vi "GUI_BELLA_StageMegattentuator.vi"() -> ()   [LabVIEW 2020]
uses:
  Shared/GUI_Template/GUI_master/tcp_new_data_event.ctl
  Shared/GUI_Template/GUI_master/tcp new data cluster.ctl
panel:
  in  "Lock Control":bool
  in  "Change Position":bool
  out "Current Status":string
  in  "stop":bool
  in  "Position.Ch1::1":dbl=0.5 caption="Current Position" min=0.0 max=150.0 format="%_4f"
  out "error IO 2":errorcluster
  out "tcp data event":T1
  in  "GUIdevice 1":string="STAGE-LT-Megattenuator"
  in  "insert tag":bool=TRUE
  # "GUI_BELLA_StageMegattentuator"
  # "IN"
  # "OUT"
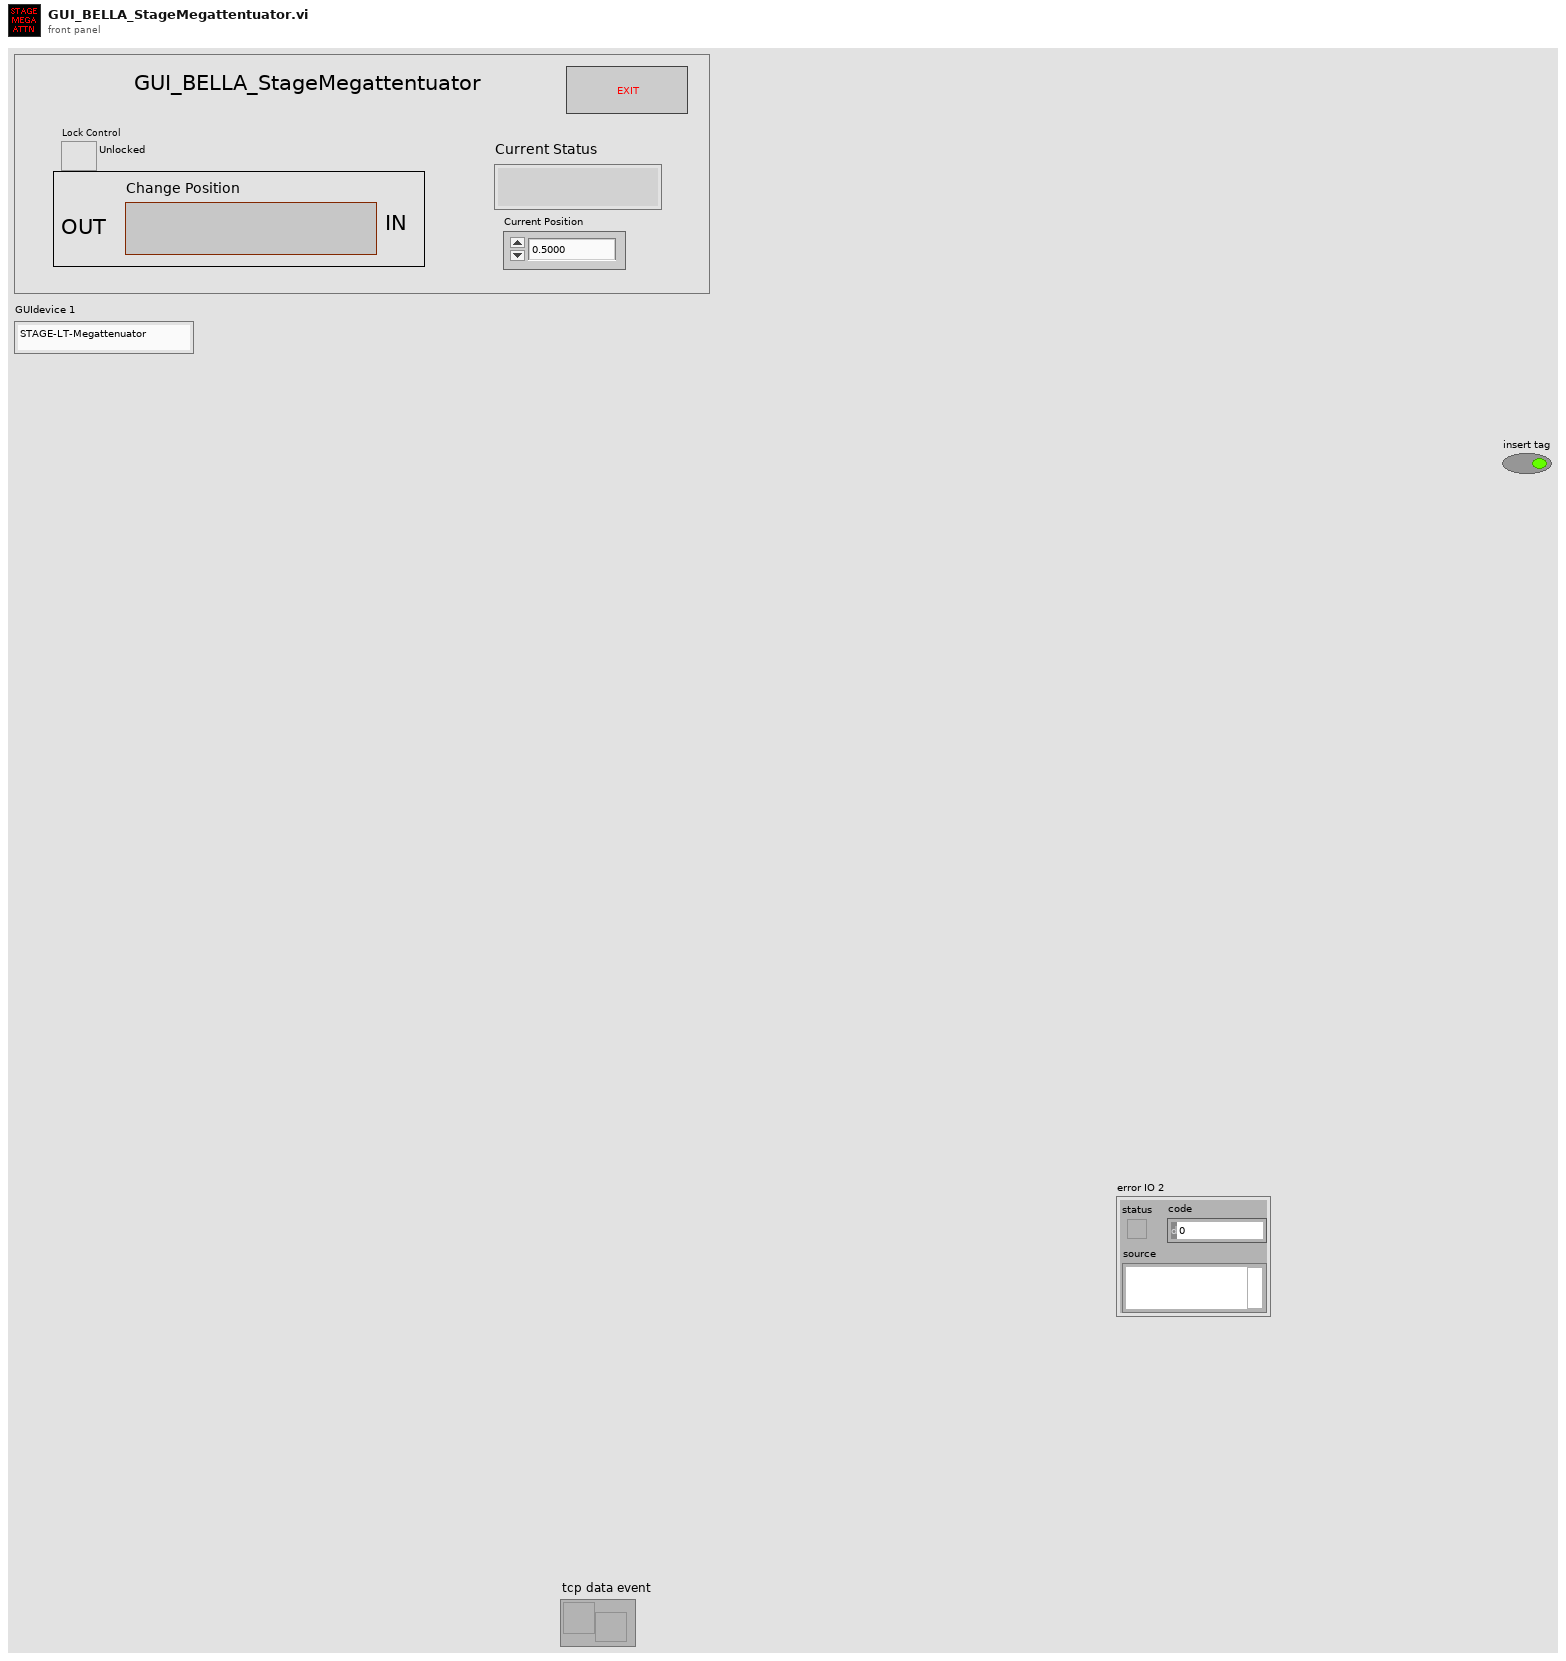
[diagram p1: front panel]
types:
  T1 = typedef "tcp_new_data_event.ctl" = refnum<user-event>
  T2 = typedef "tcp new data cluster.ctl" = cluster{"EventEnum":enum16{"new data", "connection status update"}, "Device name":string}
  T3 = enum8{"Enabled", "Disabled", "Disabled and Grayed Out"}
  T4 = enum32{"Invalid", "Standard", "Closed", "Hidden", "Minimized", "Maximized"}
  T5 = enum32{"invalid app kind", "Development System", "Run Time System", "Student Edition", "Embedded LabVIEW", "Evaluation", "Custom"}
  T6 = cluster{"Core":cluster{"Current VI Reference":refnum<vi>, "Close Panel on Exit?":bool}, "Your Boolean data":bool, "Your string data":string}
  T7 = cluster{"Current VI Reference":refnum<vi>, "Close Panel on Exit?":bool}
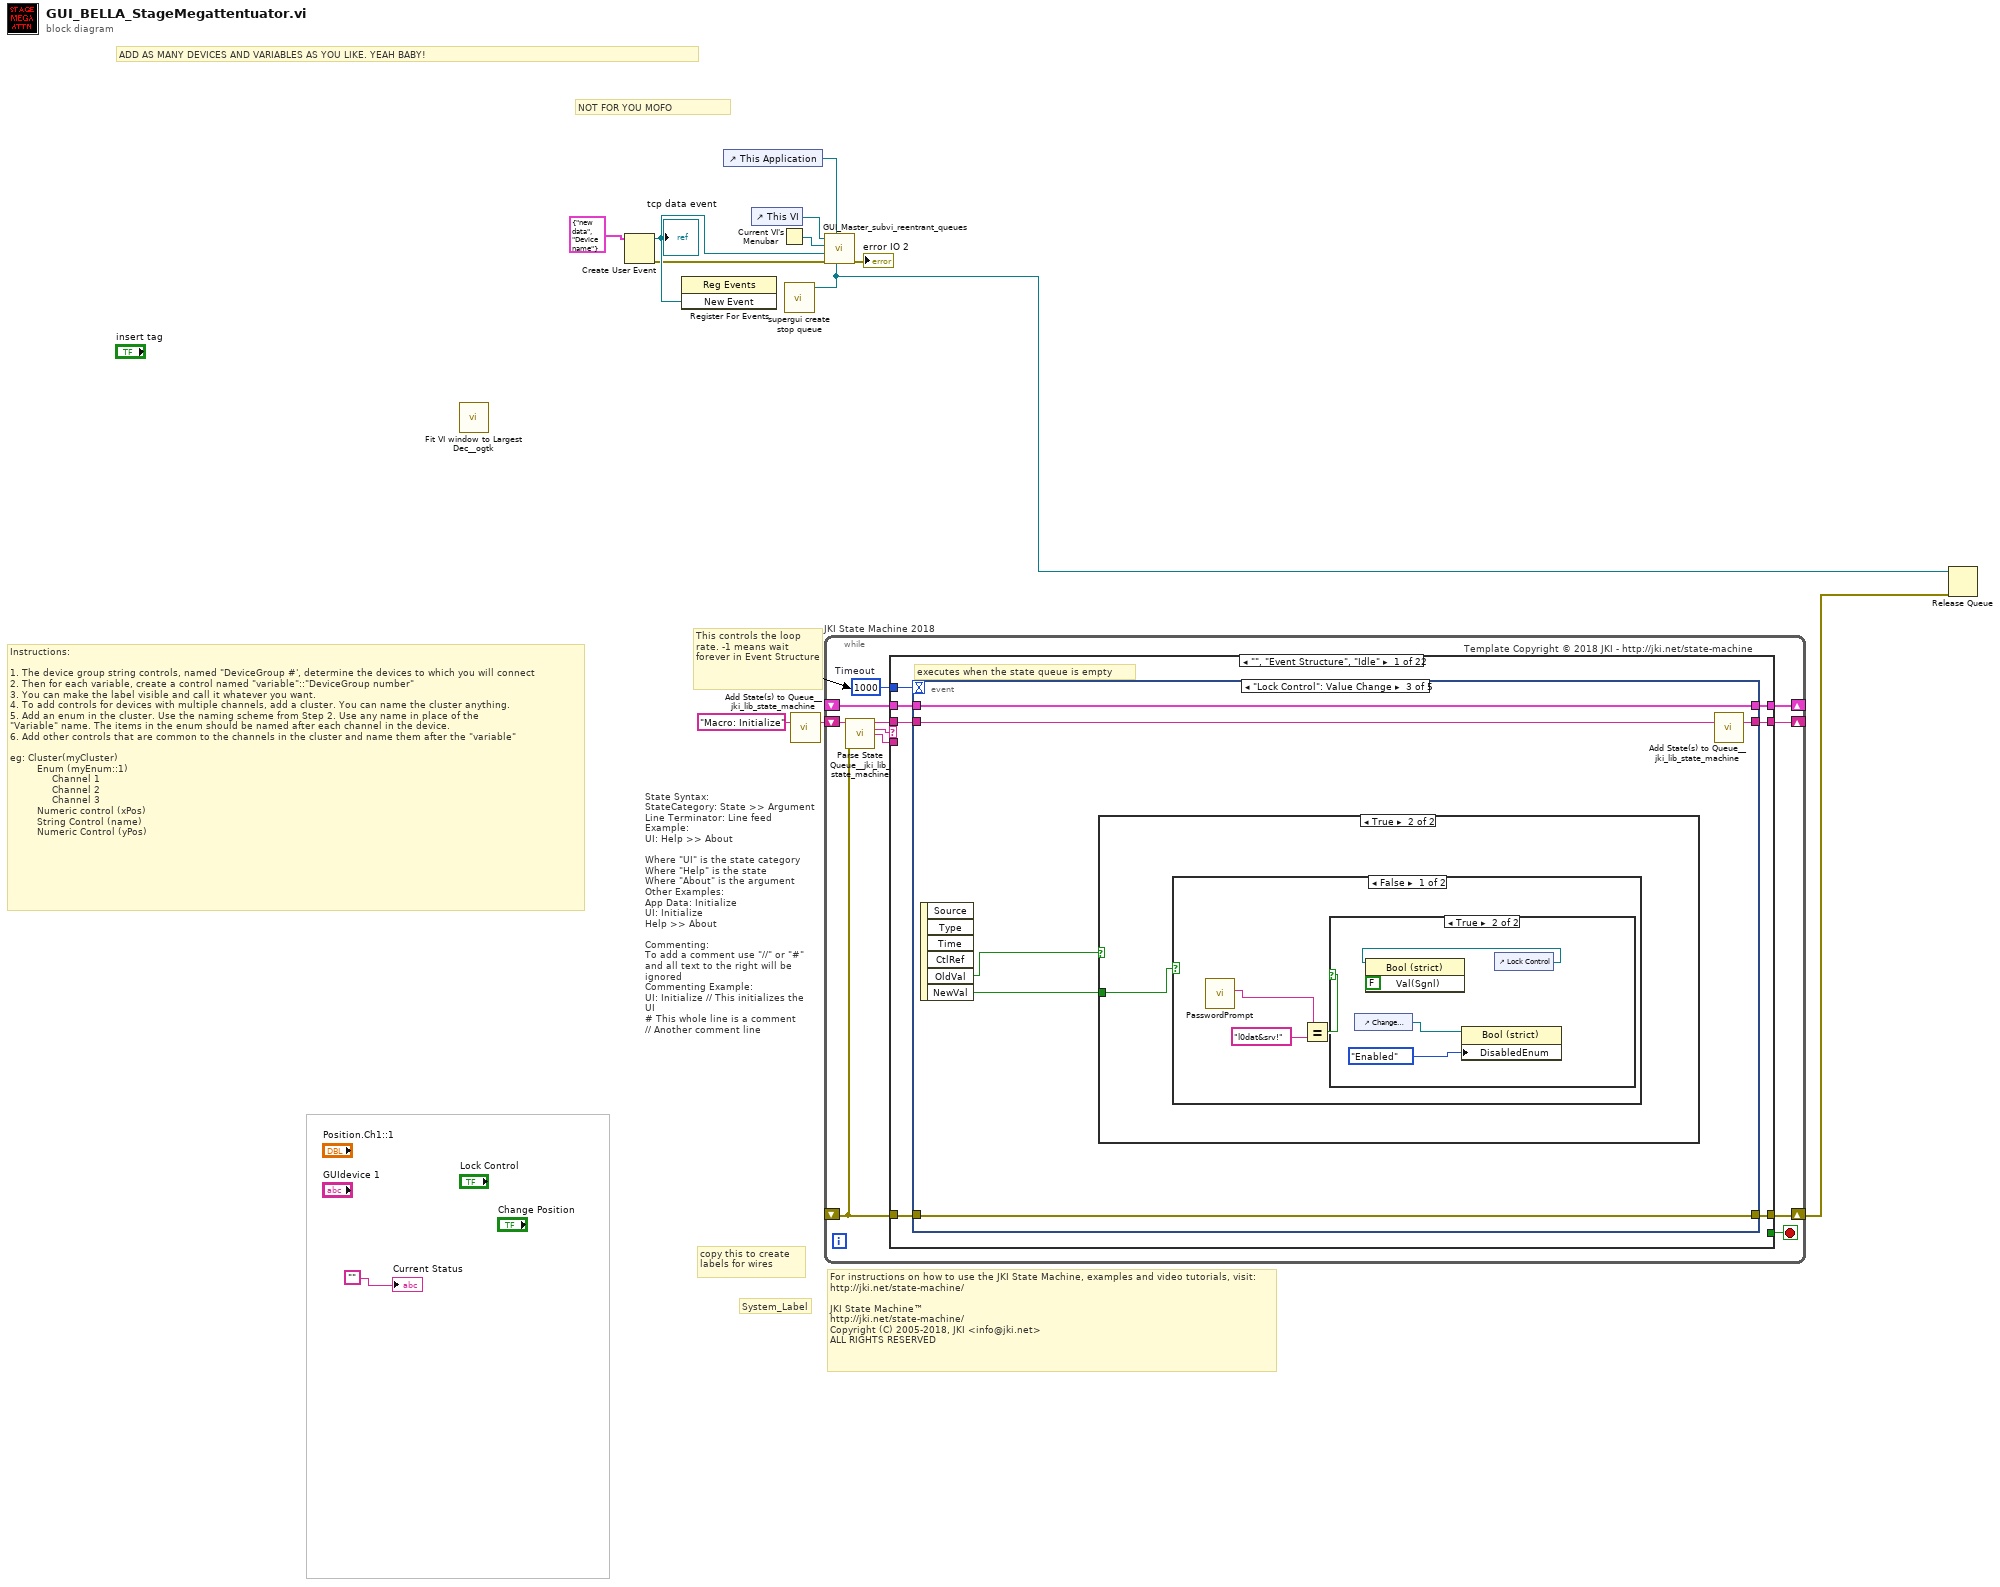
[diagram p0: block diagram]
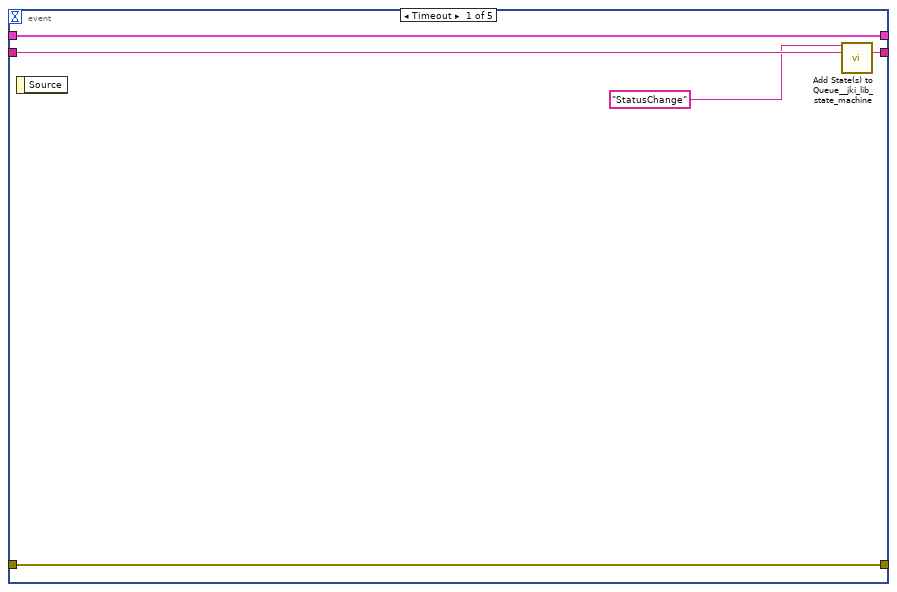
[diagram p2: hidden frame]
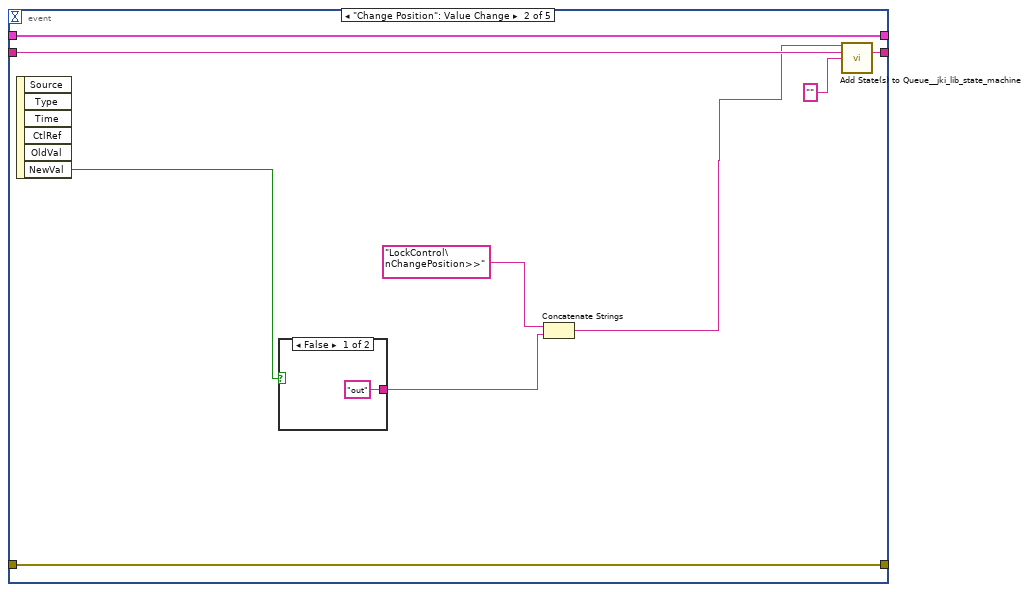
[diagram p3: hidden frame]
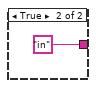
[diagram p4: hidden frame]
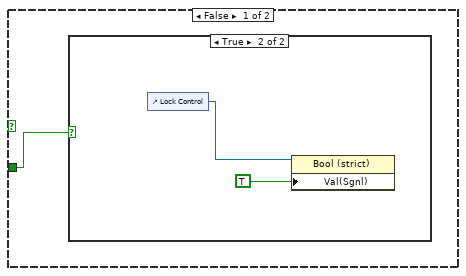
[diagram p5: hidden frame]
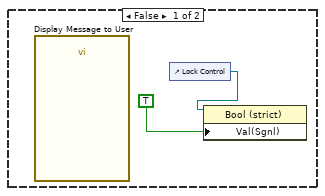
[diagram p7: hidden frame]
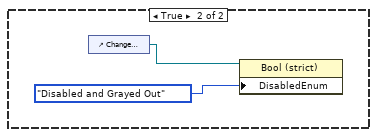
[diagram p8: hidden frame]
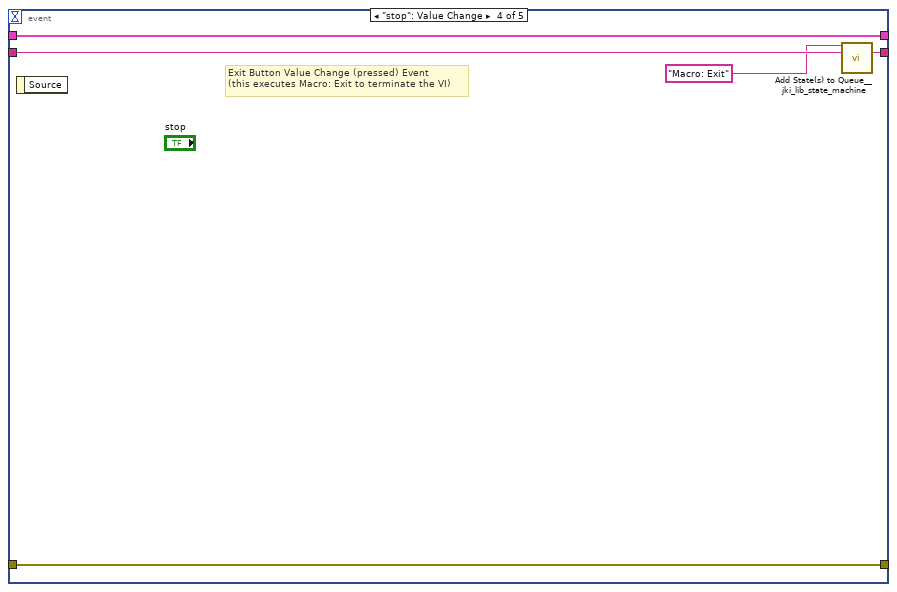
[diagram p9: hidden frame]
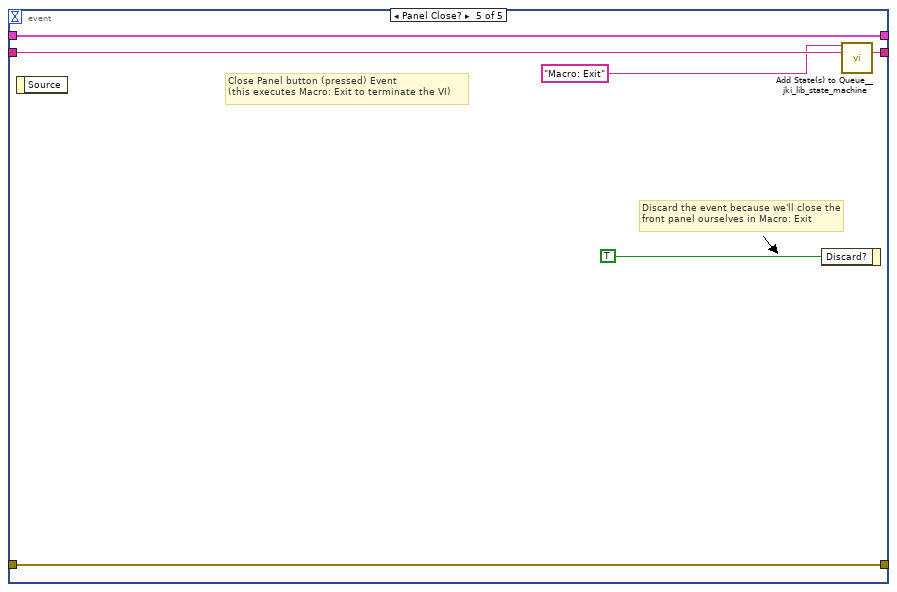
[diagram p10: hidden frame]
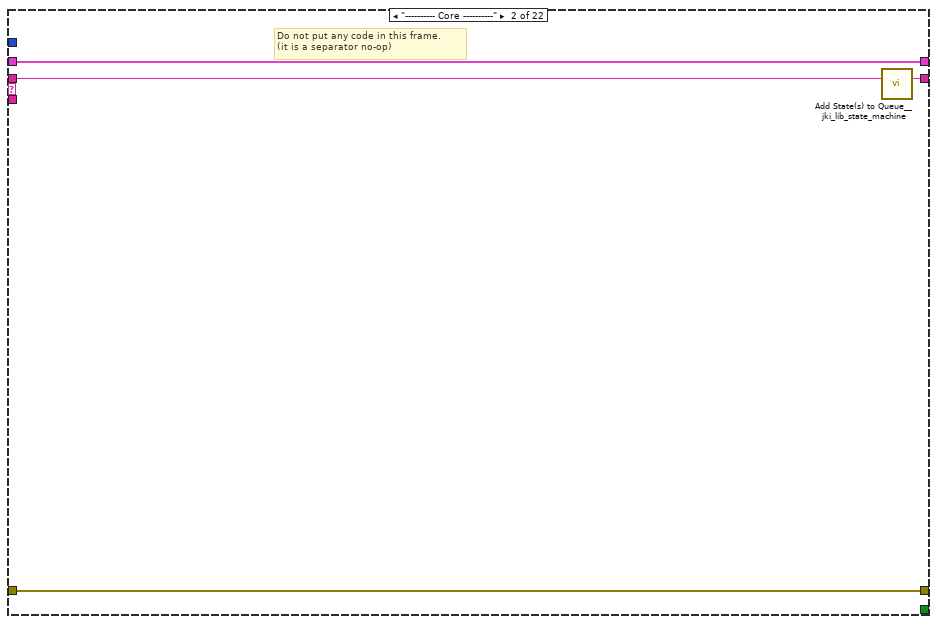
[diagram p11: hidden frame]
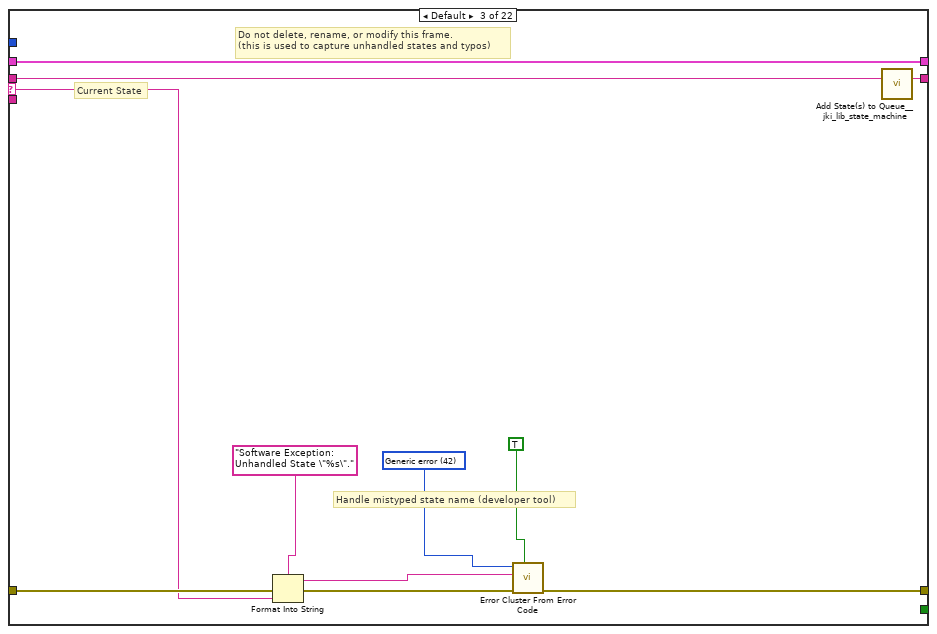
[diagram p12: hidden frame]
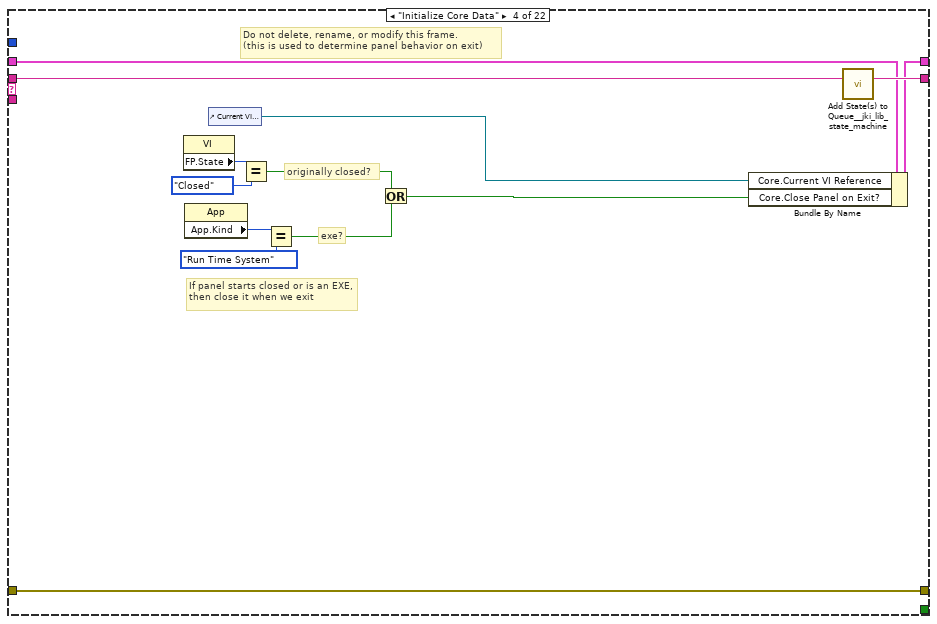
[diagram p13: hidden frame]
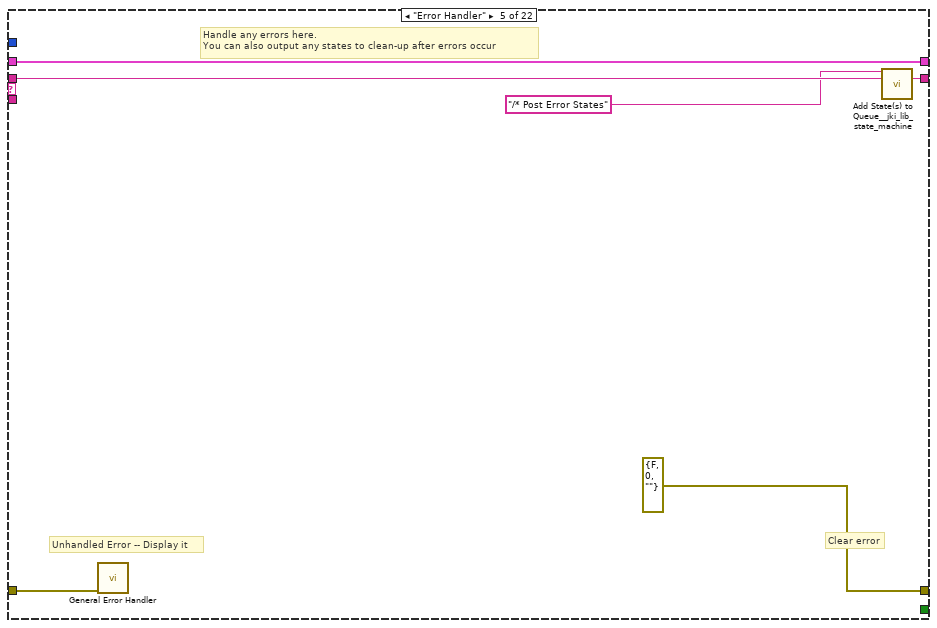
[diagram p14: hidden frame]
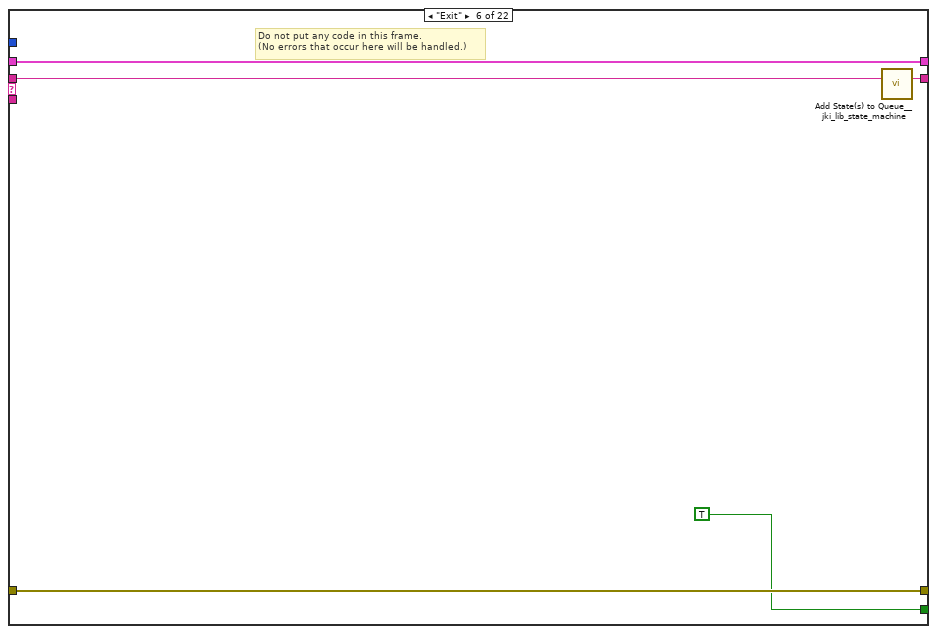
[diagram p15: hidden frame]
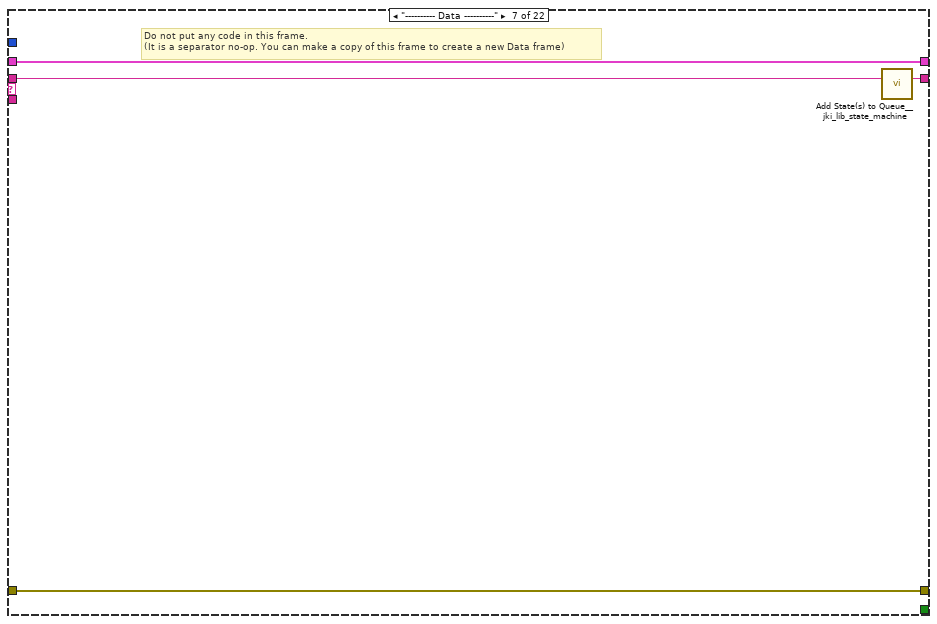
[diagram p16: hidden frame]
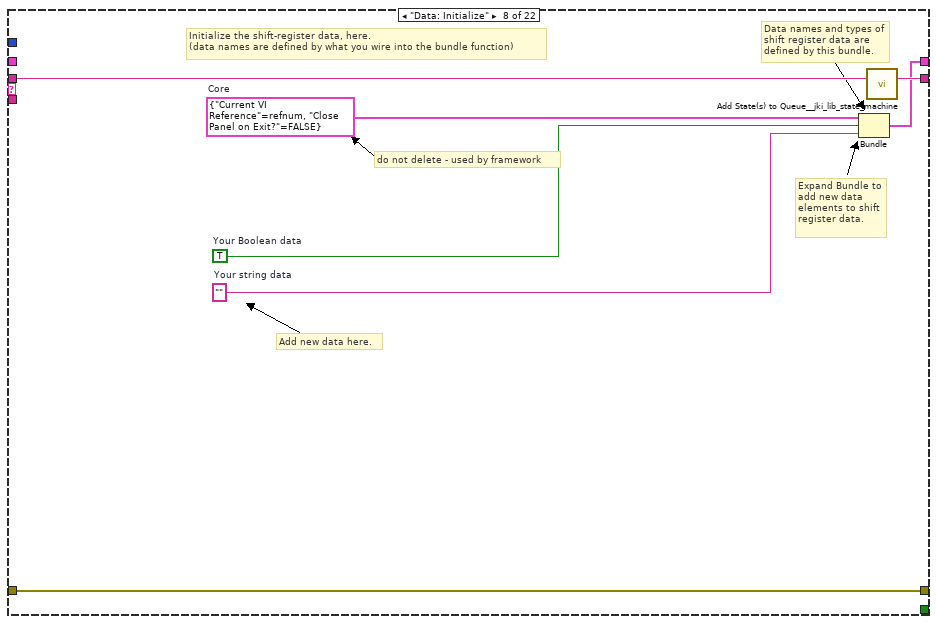
[diagram p17: hidden frame]
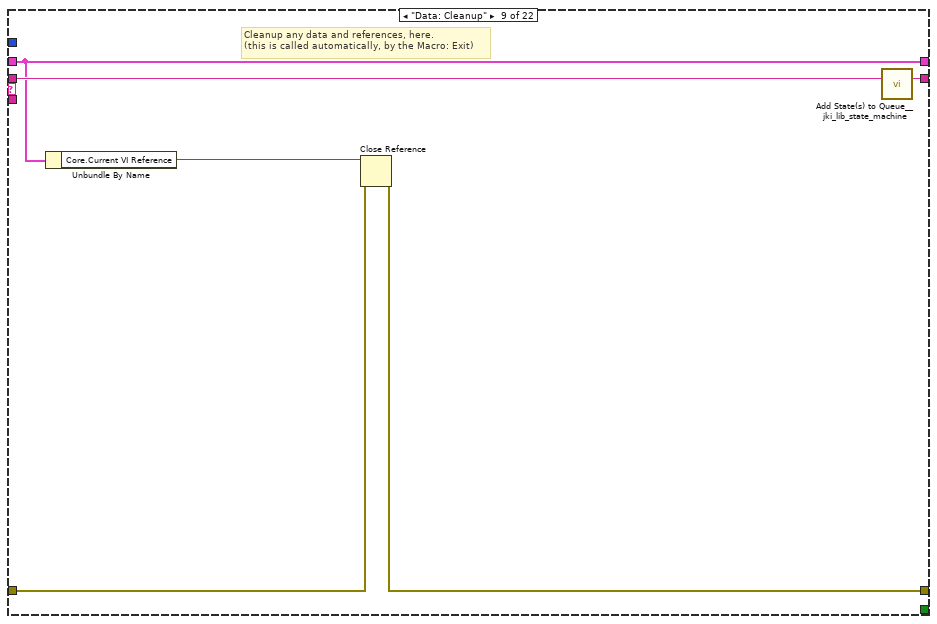
[diagram p18: hidden frame]
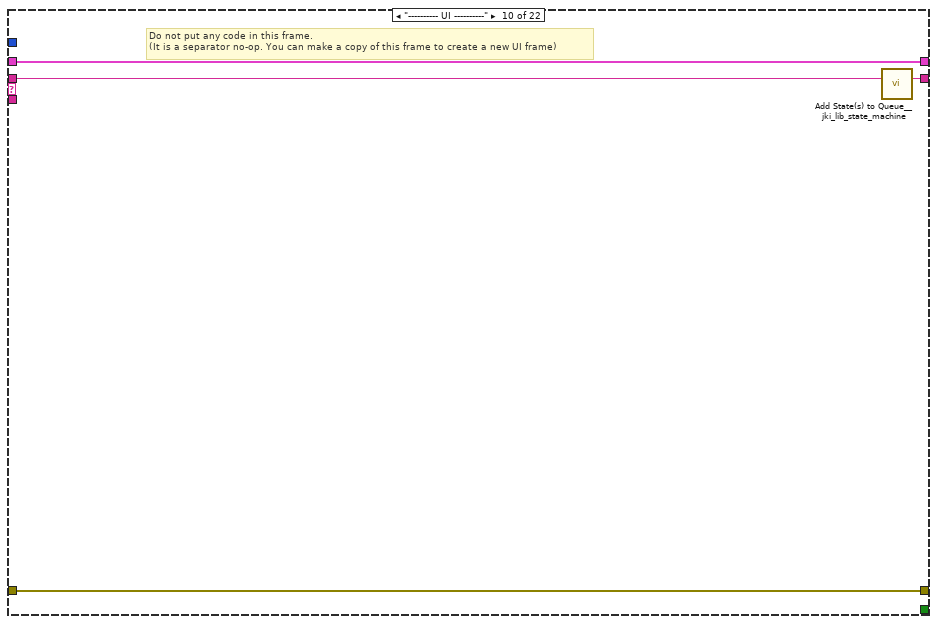
[diagram p19: hidden frame]
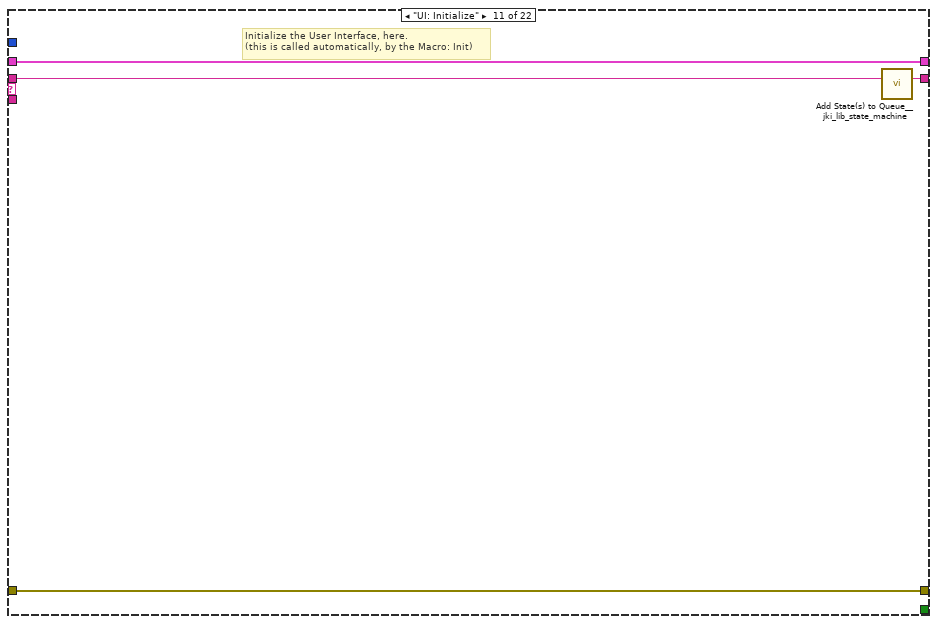
[diagram p20: hidden frame]
diagram:
  # "For instructions on how to use the JKI State Machine, examples and video tutorials, visit:\nhttp://jki.net/state-machine/\n\nJKI State Machine™\nhttp://jki.net/state-machine/\nCopyright (C) 2005-2018, JKI <info@jki.net>\nALL RIGHTS RESERVED"
  # "State Syntax:\nStateCategory: State >> Argument\nLine Terminator: Line feed\nExample:\nUI: Help >> About\n\nWhere \"UI\" is the state category\nWhere \"Help\" is the state\nWhere \"About\" is the argument\nOther Examples:\nApp Data: Initialize\nUI: Initialize\nHelp >> About\n\nCommenting:\nTo add a comment use \"//\" or \"#\" and all text to the right will be ignored\nCommenting Example:\nUI: Initialize // This initializes the UI\n# This whole line is a comment\n// Another comment line"
  # "copy this to create labels for wires"
  # "This controls the loop rate. -1 means wait forever in Event Structure"
  # "System_Label"
  # "NOT FOR YOU MOFO"
  # "Instructions:\n\n1. The device group string controls, named \"DeviceGroup #', determine the devices to which you will connect\n2. Then for each variable, create a control named \"variable\"::\"DeviceGroup number\"\n3. You can make the label visible and call it whatever you want.\n4. To add controls for devices with multiple channels, add a cluster. You can name the cluster anything.\n5. Add an enum in the cluster. Use the naming scheme from Step 2. Use any name in place of the \n\"Variable\" name. The items in the enum should be named after each channel in the device. \n6. Add other controls that are common to the channels in the cluster and name them after the \"variable\"\n\neg: Cluster(myCluster)\n         Enum (myEnum::1)\n              Channel 1 \n              Channel 2\n              Channel 3\n         Numeric control (xPos)\n         String Control (name)\n         Numeric Control (yPos)"
  # "ADD AS MANY DEVICES AND VARIABLES AS YOU LIKE. YEAH BABY!"
  n1 = call <userlib>:"Fit VI window to Largest Dec__ogtk.vi"() -> ()  [unwired: 6 in, 2 out]
  n2 = Create User Event(user event datatype=T2 {"EventEnum"=enum."new data", "Device name"="Device name"} ("New Event")) -> (user event=w11:refnum<user-event>, error out=w10:errorcluster)  [unwired: 1 in]
  "tcp data event" <- w11
  n3 = register-events(w11) -> ()  [unwired: 2 in, 2 out]
  n4 = control-ref of="This Application"() -> (w12:refnum<vi>)
  n5 = control-ref of="This VI"() -> (w7:refnum<vi>)
  n6 = Current VI's Menubar() -> (w8:refnum<k9>)
  n7 = call "supergui create stop queue.vi"() -> ("STOP Queue out"=w5:refnum<queue>)  [unwired: 11 in]
  n8 = call <vilib>:"Add State(s) to Queue__jki_lib_state_machine.vi"("State(s) in (\"\")"="Macro: Initialize") -> ("States Out"=w4:string)  [unwired: 14 in]
  n9 = call "GUI_Master_subvi_reentrant_queues.vi"("STOP Queue in"=w5, "This Application"=w12, "error in (no error)"=w10, "tcp data event"=w11, "Caller menu reference"=w8, "Caller VI ref"=w7) -> ("error out"=→"error IO 2":errorcluster)  [unwired: 5 in]
  n10 = while "JKI State Machine 2018" {
    shift-right: [w16] -> _
    shift-left: _ -> [w15]
    shift-right: [w19] -> w2
    shift-left: _ -> [w13]
    shift-right: [w18] -> _
    shift-left: w4 -> [w20]
    stop <- w17 stop-if-true
    w14 = 1000  # Timeout
    # "Template Copyright © 2018 JKI - http://jki.net/state-machine"
    n11 = call <vilib>:"Parse State Queue__jki_lib_state_machine.vi"("State Queue"=w20, "Error In (no error)"=w13) -> ("Remaining States"=w22:string, "Current State"=w23:string, "Arguments"=w21:string)  [unwired: 11 in]
    n12 = case shown="\"\", \"Event Structure\", \"Idle\"" w23 {
      selector: w23 -> [_ _ w83 _ _ _ _ _ _ _ _ _ _ _ _ _ _ _ _ _ _ _]
      tunnel: w22 -> [w30 w82 w87 w106 w112 w117 w121 w128 w134 w138 w142 w148 w159 w228 w233 w243 w247 w252 w262 w269 w280 w285]
      tunnel: w21 -> [_ _ _ _ _ _ _ _ _ _ _ w143 w153 _ _ _ _ w248 _ _ _ _]
      tunnel: w15 -> [w28 w79 w85 w99 w109 w115 w118 _ w129 w135 w140 w146 w155 w225 w230 w240 w244 w249 w259 w266 w277 w282]
      tunnel: [w27 w80 w89 w103 errorcluster {"status"=FALSE, "code"=0, "source"=""} ("error out") w114 w119 w125 w130 w136 w139 w144 w156 w226 w231 w241 w245 w250 w260 w267 w278 w283] -> w19
      tunnel: w13 -> [w26 w80 w88 w103 w108 w114 w119 w125 w131 w136 w139 w145 w157 w226 w231 w241 w245 w250 w260 w267 w278 w283]
      tunnel: [w29 w81 w86 w105 w111 w116 w120 w127 w133 w137 w141 w147 w158 w227 w232 w242 w246 w251 w261 w268 w279 w284] -> w18
      tunnel: [_ _ _ _ _ TRUE _ _ _ _ _ _ _ _ _ _ _ _ _ _ _ _] -> w17
      tunnel: [w25 w79 w85 w104 w109 w115 w118 w126 w129 w135 w140 w146 w155 w225 w230 w240 w244 w249 w259 w266 w277 w282] -> w16
      tunnel: w14 -> [w24 _ _ _ _ _ _ _ _ _ _ _ _ _ _ _ _ _ _ _ _ _]
      frame "", "Event Structure", "Idle" {
        # "executes when the state queue is empty"
        n13 = event shown="[2] \"Lock Control\": Value Change" {
          selector: _ -> [_ _ _ _ _]
          dyn-events: _ -> [_ _ _ _ _]
          timeout: w24 -> [_ _ _ _ _]
          tunnel: w30 -> [w35 w44 w52 w72 w78]
          tunnel: [w34 w43 w51 w71 w77] -> w29
          tunnel: w28 -> [w32 w41 w49 w69 w75]
          tunnel: [w33 w42 w50 w70 w76] -> w27
          tunnel: w26 -> [w33 w42 w50 w70 w76]
          tunnel: [w32 w41 w49 w69 w75] -> w25
          event Timeout {
            n14 = event-data() -> ()  [unwired: 1 in, 1 out]
            n15 = call <vilib>:"Add State(s) to Queue__jki_lib_state_machine.vi"("State(s) in Front (\"\")"="StatusChange" ("State(s) in Front (\"\")"), "State(s) in (\"\")"=w35) -> ("States Out"=w34:string)  [unwired: 13 in]
          }
          event "Change Position": Value Change {
            n16 = event-data() -> ("NewVal"=w38:bool)  [unwired: 1 in, 5 out]
            n17 = case shown="False" w38 {
              tunnel: ["out" "in"] -> w39
              frame False {
              }
              frame True {
              }
            }
            n18 = Concatenate Strings("LockControl\nChangePosition>>" ("State(s) in Front (\"\")"), w39) -> (w37:string)
            n19 = call <vilib>:"Add State(s) to Queue__jki_lib_state_machine.vi"("State(s) in Front (\"\")"=w37, "State(s) in (\"\")"=w44, "State(s) at Back (\"\")"="" ("State(s) at Back (\"\")")) -> ("States Out"=w43:string)  [unwired: 12 in]
          }
          event "Lock Control": Value Change {
            n20 = event-data() -> ("OldVal"=w48:bool, "NewVal"=w47:bool)  [unwired: 1 in, 4 out]
            n21 = case shown="True" w48 {
              tunnel: w47 -> [w53 w56]
              frame False {
                n22 = case shown="True" w53 {
                  frame False {
                  }
                  frame True {
                    n23 = control-ref of="Lock Control"() -> (w54:refnum<vi>)
                    n24 = property on="Property Node" class="Bool (strict)"(reference=w54, "Val(Sgnl)"=TRUE ("Value (Signaling)")) -> ()  [unwired: 1 in, 2 out]
                  }
                }
              }
              frame True {
                n25 = case shown="False" w56 {
                  frame False {
                    n26 = call "PasswordPrompt.vi"() -> ("Please enter password below 2"=w57:string)  [unwired: 11 in]
                    n27 = Equal?(x=w57, y="l0dat&srv!") -> (x = y?=w59:bool)
                    n28 = case shown="True" w59 {
                      frame False {
                        n29 = call "Display Message to User"() -> ()  [unwired: 10 in, 2 out]
                        n30 = control-ref of="Lock Control"() -> (w60:refnum<vi>)
                        n31 = property on="Property Node" class="Bool (strict)"(reference=w60, "Val(Sgnl)"=TRUE ("Value (Signaling)")) -> ()  [unwired: 1 in, 2 out]
                      }
                      frame True {
                        n32 = control-ref of="Change Position"() -> (w62:refnum<vi>)
                        n33 = property on="Property Node" class="Bool (strict)"(reference=w62, "DisabledEnum"=T3."Enabled" ("Disabled")) -> ()  [unwired: 1 in, 2 out]
                        n34 = control-ref of="Lock Control"() -> (w63:refnum<vi>)
                        n35 = property on="Property Node" class="Bool (strict)"(reference=w63, "Val(Sgnl)"=FALSE ("Value (Signaling)")) -> ()  [unwired: 1 in, 2 out]
                      }
                    }
                  }
                  frame True {
                    n36 = control-ref of="Change Position"() -> (w66:refnum<vi>)
                    n37 = property on="Property Node" class="Bool (strict)"(reference=w66, "DisabledEnum"=T3."Disabled and Grayed Out" ("Disabled")) -> ()  [unwired: 1 in, 2 out]
                  }
                }
              }
            }
            n38 = call <vilib>:"Add State(s) to Queue__jki_lib_state_machine.vi"("State(s) in (\"\")"=w52) -> ("States Out"=w51:string)  [unwired: 14 in]
          }
          event "stop": Value Change {
            # "Exit Button Value Change (pressed) Event\n(this executes Macro: Exit to terminate the VI)"
            n39 = event-data() -> ()  [unwired: 1 in, 1 out]
            n40 = call <vilib>:"Add State(s) to Queue__jki_lib_state_machine.vi"("State(s) in Front (\"\")"="Macro: Exit", "State(s) in (\"\")"=w72) -> ("States Out"=w71:string)  [unwired: 13 in]
          }
          event Panel Close? {
            # "Discard the event because we'll close the front panel ourselves in Macro: Exit"
            # "Close Panel button (pressed) Event\n(this executes Macro: Exit to terminate the VI)"
            n41 = event-data() -> ()  [unwired: 1 in, 1 out]
            n42 = event-data("Discard?"=TRUE) -> ()  [unwired: 1 in, 1 out]
            n43 = call <vilib>:"Add State(s) to Queue__jki_lib_state_machine.vi"("State(s) in Front (\"\")"="Macro: Exit", "State(s) in (\"\")"=w78) -> ("States Out"=w77:string)  [unwired: 13 in]
          }
        }
      }
      frame "---------- Core ----------" {
        # "Do not put any code in this frame.\n(it is a separator no-op)"
        n44 = call <vilib>:"Add State(s) to Queue__jki_lib_state_machine.vi"("State(s) in (\"\")"=w82) -> ("States Out"=w81:string)  [unwired: 14 in]
      }
      frame Default {
        w92 = 42 items=["No error", "Argument error", "Memory is full", "Out of zone", "End of file", "File already open", "Generic file I/O error", "File not found", "File permission error", "Disk is full", "Duplicate path", "Too many files open", "System feature not enabled", "Resource file not found", "Cannot add resource", "Resource not found", "Image not found", "Image memory error", "Pen does not exist", "Config type invalid", "Config token not found", "Config parse error", "Config memory error", "Bad external code format", "Bad external code offset", "External code not present", "Null window", "Destroy window error", "Null menu", "Print aborted", "Bad print record", "Print driver error", "Windows error during printing", "Memory error during printing", "Print dialog error", "Generic print error", "Invalid device refnum", "Device not found", "Device parameter error", "Device unit error", "Cannot open device", "Device call aborted", "Generic error", "Cancelled by user", "Object ID too low", "Object ID too high", "Object not in heap", "Unknown heap", "Unknown object (invalid DefProc)", "Unknown object (DefProc not in table)", "Message out of range", "Invalid (null) method", "Unknown message", "Manager call not supported", "Bad address", "Network operation in progress", "Network operation timed out", "Connection is busy", "Network attribute not supported", "Network error", "Address in use", "System out of memory", "Connection aborted", "Connection refused", "Not connected", "Already connected", "Connection closed", "Initialization error (interapplication manager)", "Bad occurrence", "Wait on unbound occurrence handler", "Occurrence queue overflow", "Datalog type conflict", "Unused", "Unrecognized type (interapplication manager)", "Memory corrupt", "Failed to make temporary DLL", "Old CIN version", "Drag socket not found", "Failed to load drop-object", "Failed to register OLE object", "Failed to release OLE object", "Format specifier type mismatch", "Unknown format specifier", "Too few format specifiers", "Too many format specifiers", "Scan failed", "Newer CIN version", "Error converting to variant", "Runtime menu error", "Password tampered", "Variant attribute not found", "Incompatible variant data type", "Event data is not available", "Event Store is not present", "Occurrence is not found", "Event Queue is not created", "Event info is not available", "Refnum passed is NULL", "Error retrieving Class GUID", "Error retrieving CoClass GUID", "Error retrieving TypeLib GUID.", "Bad built application magic bytes.", "Specific driver is different from the specific driver associated with the Logical Name.", "There is no session opened to the class driver.", "Max Error", "MAX - Error with config objects", "MAX - Error loading configuration", "MAX - Group not supported"]
        # "Current State"
        # "Do not delete, rename, or modify this frame.\n(this is used to capture unhandled states and typos)"
        # "Handle mistyped state name (developer tool)"
        n45 = Format Into String(format string="Software Exception: Unhandled State \"%s\"." ("message"), error in=w88, w83) -> (resulting string=w91:string, error out=w90:errorcluster)  [unwired: 1 in]
        n46 = call <vilib>:"Error Cluster From Error Code.vi"("show call chain? (False)"=TRUE, "error in (no error)"=w90, "error message (\"\")"=w91, "error code (0)"=w92) -> ("error out"=w89:errorcluster)  [unwired: 5 in]
        n47 = call <vilib>:"Add State(s) to Queue__jki_lib_state_machine.vi"("State(s) in (\"\")"=w87) -> ("States Out"=w86:string)  [unwired: 14 in]
      }
      frame "Initialize Core Data" {
        # "Do not delete, rename, or modify this frame.\n(this is used to determine panel behavior on exit)"
        # "originally closed?"
        # "exe?"
        # "If panel starts closed or is an EXE, then close it when we exit"
        n48 = property class="VI"() -> ("FP.State"=w96:T4)  [unwired: 2 in, 2 out]
        n49 = property class="App"() -> ("App.Kind"=w102:T5)  [unwired: 2 in, 2 out]
        n50 = control-ref of="Current VI Reference"() -> (w97:refnum<vi>)
        n51 = Equal?(x=w96, y=T4."Closed" ("Front Panel Window:State")) -> (x = y?=w94:bool)
        n52 = Equal?(x=w102, y=T5."Run Time System" ("Application:Kind")) -> (x = y?=w100:bool)
        n53 = Or(x=w94, y=w100) -> (x .or. y?=w98:bool)
        n54 = Bundle By Name(cluster=w99, "Core.Current VI Reference"=w97, "Core.Close Panel on Exit?"=w98) -> (w104:T6)
        n55 = call <vilib>:"Add State(s) to Queue__jki_lib_state_machine.vi"("State(s) in (\"\")"=w106) -> ("States Out"=w105:string)  [unwired: 14 in]
      }
      frame "Error Handler" {
        # "Unhandled Error -- Display it"
        # "Handle any errors here.\nYou can also output any states to clean-up after errors occur"
        # "Clear error"
        n56 = call <vilib>:"General Error Handler.vi"("error in (no error)"=w108) -> ()  [unwired: 10 in, 5 out]
        n57 = call <vilib>:"Add State(s) to Queue__jki_lib_state_machine.vi"("State(s) in Front (\"\")"="/* Post Error States", "State(s) in (\"\")"=w112) -> ("States Out"=w111:string)  [unwired: 13 in]
      }
      frame "Exit" {
        # "Do not put any code in this frame.\n(No errors that occur here will be handled.)"
        n58 = call <vilib>:"Add State(s) to Queue__jki_lib_state_machine.vi"("State(s) in (\"\")"=w117) -> ("States Out"=w116:string)  [unwired: 14 in]
      }
      frame "---------- Data ----------" {
        # "Do not put any code in this frame.\n(It is a separator no-op. You can make a copy of this frame to create a new Data frame)"
        n59 = call <vilib>:"Add State(s) to Queue__jki_lib_state_machine.vi"("State(s) in (\"\")"=w121) -> ("States Out"=w120:string)  [unwired: 14 in]
      }
      frame "Data: Initialize" {
        w122 = T7 {"Current VI Reference"=refnum, "Close Panel on Exit?"=FALSE}  # Core
        w124 = TRUE  # Your Boolean data
        w123 = ""  # Your string data
        # "do not delete - used by framework"
        # "Expand Bundle to add new data elements to shift register data."
        # "Add new data here."
        # "Data names and types of shift register data are defined by this bundle."
        # "Initialize the shift-register data, here.\n(data names are defined by what you wire into the bundle function)"
        n60 = Bundle("Core"=w122, "Your Boolean data"=w124, "Your string data"=w123) -> (w126:T6)  [unwired: 1 in]
        n61 = call <vilib>:"Add State(s) to Queue__jki_lib_state_machine.vi"("State(s) in (\"\")"=w128) -> ("States Out"=w127:string)  [unwired: 14 in]
      }
      frame "Data: Cleanup" {
        # "Cleanup any data and references, here.\n(this is called automatically, by the Macro: Exit)"
        n62 = Unbundle By Name(w129) -> ("Core.Current VI Reference"=w132:refnum<vi>)
        n63 = Close Reference(reference=w132, error in (no error)=w131) -> (error out=w130:errorcluster)
        n64 = call <vilib>:"Add State(s) to Queue__jki_lib_state_machine.vi"("State(s) in (\"\")"=w134) -> ("States Out"=w133:string)  [unwired: 14 in]
      }
      frame "---------- UI ----------" {
        # "Do not put any code in this frame.\n(It is a separator no-op. You can make a copy of this frame to create a new UI frame)"
        n65 = call <vilib>:"Add State(s) to Queue__jki_lib_state_machine.vi"("State(s) in (\"\")"=w138) -> ("States Out"=w137:string)  [unwired: 14 in]
      }
      frame "UI: Initialize" {
        # "Initialize the User Interface, here.\n(this is called automatically, by the Macro: Init)"
        n66 = call <vilib>:"Add State(s) to Queue__jki_lib_state_machine.vi"("State(s) in (\"\")"=w142) -> ("States Out"=w141:string)  [unwired: 14 in]
      }
      frame "UI: Cursor Set" {
        # "Argument"
        # "Set and Unset Cursor Busy.\n(Usage: \"UI: Cursor Set >> Busy|Idle\")"
        n67 = case shown="\"Idle\", Default" w143 {
          tunnel: w145 -> [w150 w152]
          tunnel: [w149 w151] -> w144
          frame "Idle", Default {
            n68 = call <vilib>:"Unset Busy.vi"("error in (no error)"=w150) -> ("error out"=w149:errorcluster)  [unwired: 10 in]
          }
          frame "Busy" {
            n69 = call <vilib>:"Set Busy.vi"("error in (no error)"=w152) -> ("error out"=w151:errorcluster)  [unwired: 9 in, 1 out]
          }
        }
        n70 = call <vilib>:"Add State(s) to Queue__jki_lib_state_machine.vi"("State(s) in (\"\")"=w148) -> ("States Out"=w147:string)  [unwired: 14 in]
      }
      frame "UI: Front Panel State" {
        # "Argument"
        # "Set Front Panel Open or Closed\n(Usage: \"UI: Front Panel State >> Open|Close\")"
        n71 = Unbundle By Name(w155) -> ("Core.Current VI Reference"=w154:refnum<vi>)
        n72 = case shown="\"Minimize\", \"Minimized\"" w153 {
          tunnel: w157 -> [w165 w180 w191 w204 w217]
          tunnel: [w167 w181 w193 w206 w219] -> w156
          tunnel: w154 -> [w166 w178 w192 w205 w218]
          frame "Open", "Standard", Default {
            w160 = T4."Standard" ("State")
            n73 = property class="VI"(reference=w166, error in=w165) -> (reference out=w163:refnum<vi>, error out=w164:errorcluster, "FP.State"=w162:T4)
            n74 = Not Equal?(x=w162, y=w160) -> (x != y?=w161:bool)
            n75 = case shown="True" w161 {
              tunnel: [w171 w173] -> w167
              tunnel: w164 -> [w170 w173]
              tunnel: w163 -> [w169 _]
              tunnel: w160 -> [w168 _]
              frame True {
                n76 = invoke class="VI" method="FP.Open"(reference=w169, error in=w170, "Activate"=TRUE, "State"=w168) -> (error out=w171:errorcluster)  [unwired: 1 in, 4 out]
              }
              frame False {
              }
            }
          }
          frame "Close", "Closed" {
            n77 = property class="VI"(reference=w178, error in=w180) -> (reference out=w177:refnum<vi>, error out=w179:errorcluster, "FP.State"=w175:T4)
            n78 = Not Equal?(x=w175, y=T4."Closed" ("Front Panel Window:State")) -> (x != y?=w174:bool)
            n79 = case shown="True" w174 {
              tunnel: [w182 w185] -> w181
              tunnel: w179 -> [w182 w184]
              tunnel: w177 -> [_ w183]
              frame False {
              }
              frame True {
                n80 = invoke class="VI" method="FP.Close"(reference=w183, error in=w184) -> (error out=w185:errorcluster)  [unwired: 1 in, 2 out]
              }
            }
          }
          frame "Hidden", "Hide" {
            w186 = T4."Hidden" ("State")
            n81 = property class="VI"(reference=w192, error in=w191) -> (reference out=w189:refnum<vi>, error out=w190:errorcluster, "FP.State"=w188:T4)
            n82 = Not Equal?(x=w188, y=w186) -> (x != y?=w187:bool)
            n83 = case shown="True" w187 {
              tunnel: [w197 w198] -> w193
              tunnel: w190 -> [w196 w198]
              tunnel: w189 -> [w195 _]
              tunnel: w186 -> [w194 _]
              frame True {
                n84 = invoke class="VI" method="FP.Open"(reference=w195, error in=w196, "State"=w194) -> (error out=w197:errorcluster)  [unwired: 2 in, 4 out]
              }
              frame False {
              }
            }
          }
          frame "Minimize", "Minimized" {
            w199 = T4."Minimized" ("State")
            n85 = property class="VI"(reference=w205, error in=w204) -> (reference out=w202:refnum<vi>, error out=w203:errorcluster, "FP.State"=w201:T4)
            n86 = Not Equal?(x=w201, y=w199) -> (x != y?=w200:bool)
            n87 = case shown="True" w200 {
              tunnel: [w210 w211] -> w206
              tunnel: w203 -> [w209 w211]
              tunnel: w202 -> [w208 _]
              tunnel: w199 -> [w207 _]
              frame True {
                n88 = invoke class="VI" method="FP.Open"(reference=w208, error in=w209, "State"=w207) -> (error out=w210:errorcluster)  [unwired: 2 in, 4 out]
              }
              frame False {
              }
            }
          }
          frame "Maximize", "Maximized" {
            w212 = T4."Maximized" ("State")
            n89 = property class="VI"(reference=w218, error in=w217) -> (reference out=w215:refnum<vi>, error out=w216:errorcluster, "FP.State"=w214:T4)
            n90 = Not Equal?(x=w214, y=w212) -> (x != y?=w213:bool)
            n91 = case shown="True" w213 {
              tunnel: [w223 w224] -> w219
              tunnel: w216 -> [w222 w224]
              tunnel: w215 -> [w221 _]
              tunnel: w212 -> [w220 _]
              frame True {
                n92 = invoke class="VI" method="FP.Open"(reference=w221, error in=w222, "State"=w220) -> (error out=w223:errorcluster)  [unwired: 2 in, 4 out]
              }
              frame False {
              }
            }
          }
        }
        n93 = call <vilib>:"Add State(s) to Queue__jki_lib_state_machine.vi"("State(s) in (\"\")"=w159) -> ("States Out"=w158:string)  [unwired: 14 in]
      }
      frame "---------- Macro ----------" {
        # "Do not put any code in this frame.\n(It is a separator no-op. You can make a copy of this frame to create a new Macro frame)"
        n94 = call <vilib>:"Add State(s) to Queue__jki_lib_state_machine.vi"("State(s) in (\"\")"=w228) -> ("States Out"=w227:string)  [unwired: 14 in]
      }
      frame "Macro: Initialize" {
        w229 = "Data: Initialize\nInitialize Core Data\nUI: Initialize\nUI: Front Panel State >> Open\nGeneralWait\nStatusChange\nInit:ChangePositionControl\nLockControl"  # Data: Initialize Initialize Core Data UI: Initialize UI: Front Panel State >> Open GeneralWait StatusChange Init:ChangePositionControl LockControl
        # "Initialization Macro\n(This is called once, when the VI starts)"
        n95 = call <vilib>:"Add State(s) to Queue__jki_lib_state_machine.vi"("State(s) in Front (\"\")"=w229, "State(s) in (\"\")"=w233) -> ("States Out"=w232:string)  [unwired: 13 in]
      }
      frame "Macro: Exit" {
        # "Exit Macro\n(This is called once, when the VI exits)"
        n96 = Unbundle By Name(w240) -> ("Core.Close Panel on Exit?"=w239:bool)
        n97 = Select(t="UI: Front Panel State >> Close", s=w239, f="") -> (s? t:f=w236:string)
        n98 = call <vilib>:"Add State(s) to Queue__jki_lib_state_machine.vi"("State(s) in (\"\")"=w236, "State(s) at Back (\"\")"="Data: Cleanup\nExit") -> ("States Out"=w234:string)  [unwired: 13 in]
        n99 = call <vilib>:"Add State(s) to Queue__jki_lib_state_machine.vi"("State(s) in Front (\"\")"=w234, "State(s) in (\"\")"=w243) -> ("States Out"=w242:string)  [unwired: 13 in]
      }
      frame "---------- New Category ----------" {
        # "Template Separator\n(You can make a copy of, or modify, this frame)"
        n100 = call <vilib>:"Add State(s) to Queue__jki_lib_state_machine.vi"("State(s) in (\"\")"=w247) -> ("States Out"=w246:string)  [unwired: 14 in]
      }
      frame "ChangePosition" {
        # "Your code here.\n(You can make a copy of, or modify, this frame)"
        n101 = case shown="\"out\"" w248 {
          frame "out" {
            n102 = control-ref of="Position.Ch1::1"() -> (w253:refnum<vi>)
            n103 = property on="Property Node" class="DigNum (strict)"(reference=w253, "Val(Sgnl)"=150.0) -> ()  [unwired: 1 in, 2 out]
          }
          frame Default {
          }
          frame "in" {
            n104 = control-ref of="Position.Ch1::1"() -> (w255:refnum<vi>)
            n105 = property on="Property Node" class="DigNum (strict)"(reference=w255, "Val(Sgnl)"=0.5) -> ()  [unwired: 1 in, 2 out]
          }
        }
        n106 = call <vilib>:"Add State(s) to Queue__jki_lib_state_machine.vi"("State(s) in (\"\")"=w252) -> ("States Out"=w251:string)  [unwired: 14 in]
      }
      frame "StatusChange" {
        # "Your code here.\n(You can make a copy of, or modify, this frame)"
        n107 = local read "Position.Ch1::1"() -> (w258:dbl)
        n108 = case shown="2, Default" w258 {
          tunnel: ["IN" "Unkown" "OUT"] -> w257
          frame 0, 1 {
          }
          frame 2, Default {
          }
          frame 149..151 {
          }
        }
        n109 = local write "Current Status"(w257) -> ()
        n110 = call <vilib>:"Add State(s) to Queue__jki_lib_state_machine.vi"("State(s) in (\"\")"=w262) -> ("States Out"=w261:string)  [unwired: 14 in]
      }
      frame "Init:ChangePositionControl" {
        # "Your code here.\n(You can make a copy of, or modify, this frame)"
        n111 = flat-sequence {
          frame #0 {
            n112 = Wait (ms)(milliseconds to wait=u32 100) -> ()  [unwired: 1 out]
          }
          frame #1 {
            n113 = property on="Current Status" class="Str"() -> ("Value"=w271:string)  [unwired: 2 in, 2 out]
            n114 = case shown="\"OUT\"" w271 {
              tunnel: [FALSE _ TRUE] -> w272
              frame "OUT" {
              }
              frame "2", Default {
              }
              frame "IN" {
              }
            }
            n115 = local write "Change Position"(w272) -> ()
          }
        }
        n116 = call <vilib>:"Add State(s) to Queue__jki_lib_state_machine.vi"("State(s) in (\"\")"=w269) -> ("States Out"=w268:string)  [unwired: 14 in]
      }
      frame "LockControl" {
        # "Your code here.\n(You can make a copy of, or modify, this frame)"
        n117 = property on="Change Position" class="Bool (strict)"("DisabledEnum"=T3."Disabled and Grayed Out" ("Disabled")) -> ()  [unwired: 2 in, 2 out]
        n118 = property on="Lock Control" class="Bool (strict)"("Val(Sgnl)"=TRUE ("Value (Signaling)")) -> ()  [unwired: 2 in, 2 out]
        n119 = call <vilib>:"Add State(s) to Queue__jki_lib_state_machine.vi"("State(s) in (\"\")"=w280) -> ("States Out"=w279:string)  [unwired: 14 in]
      }
      frame "GeneralWait" {
        # "Your code here.\n(You can make a copy of, or modify, this frame)"
        n120 = Wait (ms)(milliseconds to wait=u32 1000) -> ()  [unwired: 1 out]
        n121 = call <vilib>:"Add State(s) to Queue__jki_lib_state_machine.vi"("State(s) in (\"\")"=w285) -> ("States Out"=w284:string)  [unwired: 14 in]
      }
    }
  }
  n122 = Release Queue(queue=w5, error in (no error)=w2) -> ()  [unwired: 1 in, 3 out]
  "Current Status" <- ""
